vi "uPublisher Publish.vi"(8 "error in (no error)":errorcluster, 10 "uMsg":refnum<class "uMsg.lvclass">, 11 "uClient_Publisher in":refnum<class "uClient_Publisher.lvclass">) -> (0 "error out":errorcluster, 3 "uClient_Publisher out":refnum<class "uClient_Publisher.lvclass">)   [LabVIEW 2023, in "uLib.lvlib" / "uClient_Publisher.lvclass"]
doc: "Publish an event to the broker.\nFor optimal performance in high-throughput streaming applications, make sure to set a valid timestamp when creating the message to be published."
uses:
  uClient_Publisher.lvclass
  uMsg/uMsg/uMsg.lvclass
  uClient_Publisher.lvclass/uClient_Publisher.ctl
  uData/uData/uData.lvclass
  uMsg/uMsg/uMsg.lvclass/uMsg.ctl
  uData/uData/uData.lvclass/uData.ctl
  uMsg/uMsg/Write Payload.vi
  uData/uData/Condition Tag Name.vi
  uData/uData/Blank Key Reserved String.vi
  uTransport/uTransport/uTransport.lvclass
  uStringManipulation/uStringManipulation/uStringManipulation.lvclass
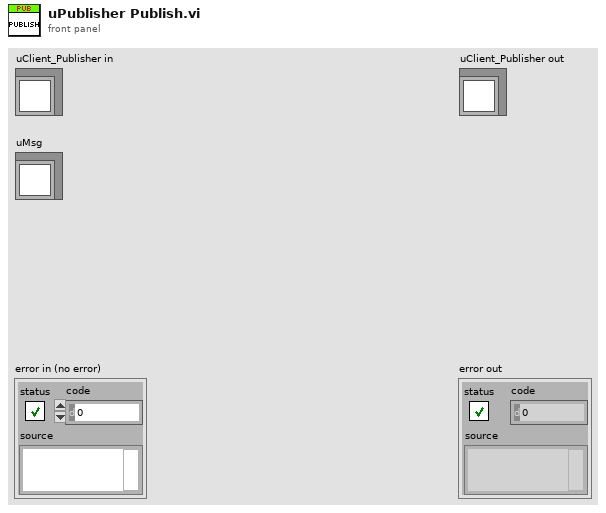
[diagram p1: front panel]
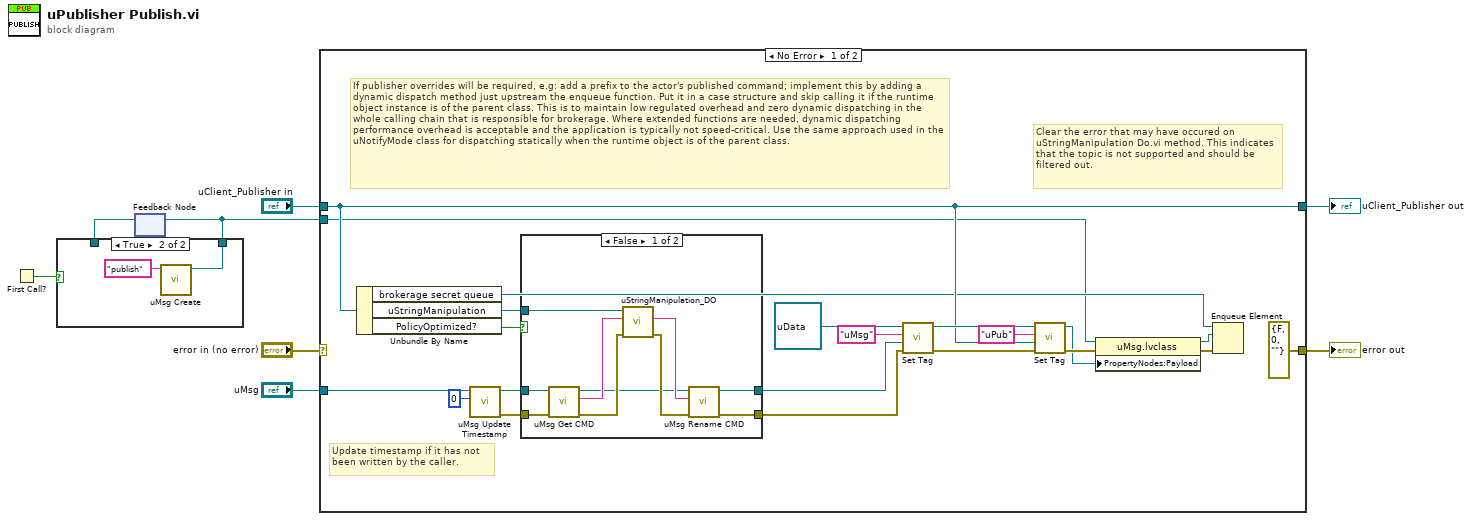
[diagram p0: block diagram]
diagram:
  n1 = First Call?() -> (First Call?: T/F=w3:bool)
  n2 = feedback #1() -> (w2:refnum<class "uMsg.lvclass">)  [unwired: 1 in]
  n3 = case shown="True" w3 {
    tunnel: [w9 w10] -> w1
    tunnel: w2 -> [w9 _]
    frame False {
    }
    frame True {
      n4 = call "uMsg Create.vi"("CMD"="publish") -> ("uMsg out"=w10:refnum<class "uMsg.lvclass">)  [unwired: 9 in, 1 out]
    }
  }
  n5 = feedback-in #1(w1) -> ()
  n6 = case shown="No Error" "error in (no error)" {
    selector: "error in (no error)" -> [_ w45]
    tunnel: [errorcluster {"status"=FALSE, "code"=0, "source"=""} ("error IO") w45] -> w8
    tunnel: "uClient_Publisher in" -> [w26 w46]
    tunnel: "uMsg" -> [w21 _]
    tunnel: [w26 w46] -> w5
    tunnel: w1 -> [w14 _]
    frame No Error {
      # "Update timestamp if it has not been written by the caller."
      # "Clear the error that may have occured on uStringManipulation Do.vi method. This indicates that the topic is not supported and should be filtered out."
      # "If publisher overrides will be required, e.g: add a prefix to the actor's published command; implement this by adding a dynamic dispatch method just upstream the enqueue function. Put it in a case structure and skip calling it if the runtime object instance is of the parent class. This is to maintain low regulated overhead and zero dynamic dispatching in the whole calling chain that is responsible for brokerage. Where extended functions are needed, dynamic dispatching performance overhead is acceptable and the application is typically not speed-critical. Use the same approach used in the uNotifyMode class for dispatching statically when the runtime object is of the parent class."
      n7 = Unbundle By Name(w26) -> ("brokerage secret queue"=w19:refnum<queue>, "uStringManipulation"=w27:refnum<class "uStringManipulation.lvclass">, "PolicyOptimized?"=w24:bool)
      n8 = call "uMsg Update Timestamp.vi"("Timestamp"=u32 0, "uMsg in"=w21) -> ("error out"=w20:errorcluster, "uMsg out"=w22:refnum<class "uMsg.lvclass">)  [unwired: 8 in]
      n9 = case shown="False" w24 {
        tunnel: w27 -> [w42 _]
        tunnel: [w41 w44] -> w18
        tunnel: w22 -> [w38 w43]
        tunnel: [w39 w43] -> w17
        tunnel: w20 -> [w34 w44]
        frame False {
          n10 = call "uMsg Get CMD.vi"("error in (no error)"=w34, "uMsg in"=w38) -> ("error out"=w37:errorcluster, "CMD"=w35:string, "uMsg out"=w33:refnum<class "uMsg.lvclass">)  [unwired: 7 in]
          n11 = call-dynamic "uStringManipulation_DO.vi"("error in (no error)"=w37, "String in"=w35, "uStringManipulation in"=w42) -> ("error out"=w36:errorcluster, "String"=w40:string)  [unwired: 6 in, 1 out]
          n12 = call "uMsg Rename CMD.vi"("error in (no error)"=w36, "New CMD"=w40, "uMsg in"=w33) -> ("error out"=w41:errorcluster, "uMsg out"=w39:refnum<class "uMsg.lvclass">)  [unwired: 7 in]
        }
        frame True {
          # "Avoid the unnecessary dynamic dispatch uStringManipulation method's overhead  if there is no translation provided."
        }
      }
      n13 = call "Set Tag.vi"("error in (no error)"=w18, "Variant"=w17, "tag (case insensitive)"="uMsg", "uData in"=refnum<class "uData.lvclass"> refnum) -> ("error out"=w32:errorcluster, "uData out"=w30:refnum<class "uData.lvclass">)  [unwired: 5 in, 1 out]
      n14 = call "Set Tag.vi"("error in (no error)"=w32, "Variant"=w26, "tag (case insensitive)"="uPub", "uData in"=w30) -> ("error out"=w16:errorcluster, "uData out"=w13:refnum<class "uData.lvclass">)  [unwired: 5 in, 1 out]
      n15 = property class="uMsg.lvclass"(reference=w14, error in=w16, "PropertyNodes:Payload"=w13) -> (reference out=w12:refnum<class "uMsg.lvclass">, error out=w15:errorcluster)
      n16 = Enqueue Element(queue=w19, element=w12, error in (no error)=w15) -> ()  [unwired: 1 in, 3 out]
    }
    frame Error {
    }
  }
  "error out" <- w8
  "uClient_Publisher out" <- w5
